vi "RVC 3-link serial robot Primatic.vi"() -> ()   [LabVIEW 2014]
uses:
  <vilib>/Analysis/Matrix/Datatypes/RealMatrix.ctl
  <vilib>/robotics/Kinematics/Analytical/Initialize Generic Serial Arm.vi
  <vilib>/robotics/Kinematics/Analytical/NI_Robotics_AnalyticKinematics.lvlib
  <vilib>/robotics/Kinematics/Robot/NI_Robotics_Serial Robot Arm.lvclass
  <vilib>/Analysis/Matrix/NI_Matrix.lvlib
panel:
  in  "appended array":dbl[](array[numeric])=[0.2, 0.2, 0.2, 0.2]
  in  "rotation angle (theta)":dbl
  in  "length (a) 2":dbl=0.3 format="%#_13g"
  in  "length (a)":dbl=0.3 format="%#_13g"
  out "transformation":picture
  out "forward kinematics":T1
  out "3D Picture":refnum<vi>(3d-picture)
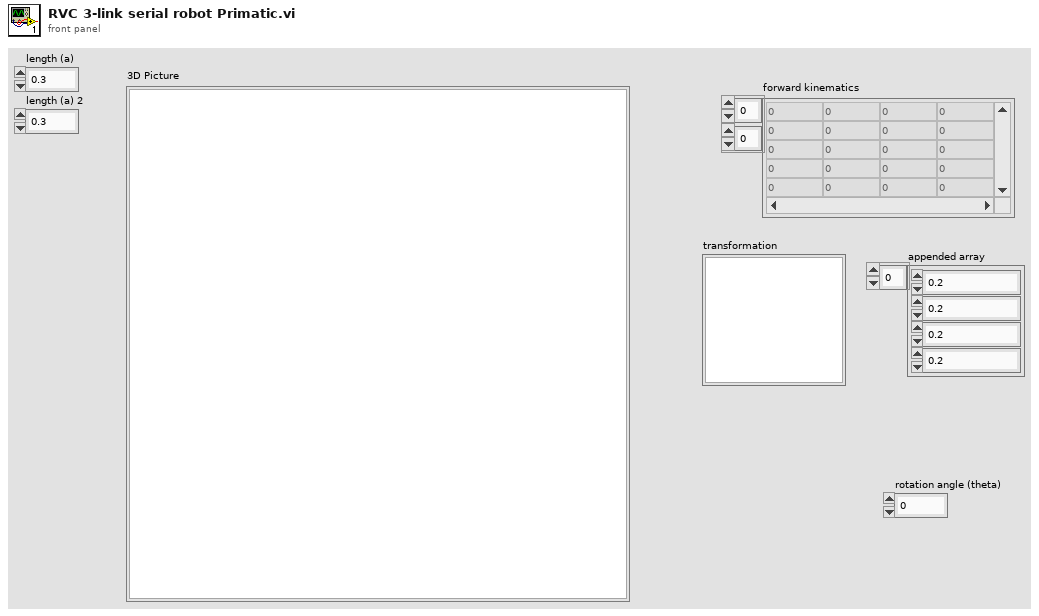
[diagram p1: front panel]
types:
  T1 = typedef "NI_Matrix.lvlib/RealMatrix.ctl" = dbl[][]
  T2 = typedef "DH Kinematic Parameters.ctl" = cluster{"twist angle":dbl, "length":dbl, "rotation angle":dbl, "offset distance":dbl, "joint type":T3, "joint coordinate offset":dbl}
  T3 = typedef "NI_Robotics_Link.lvclass/Joint Type.ctl" = enum16{"Revolute", "Prismatic"}
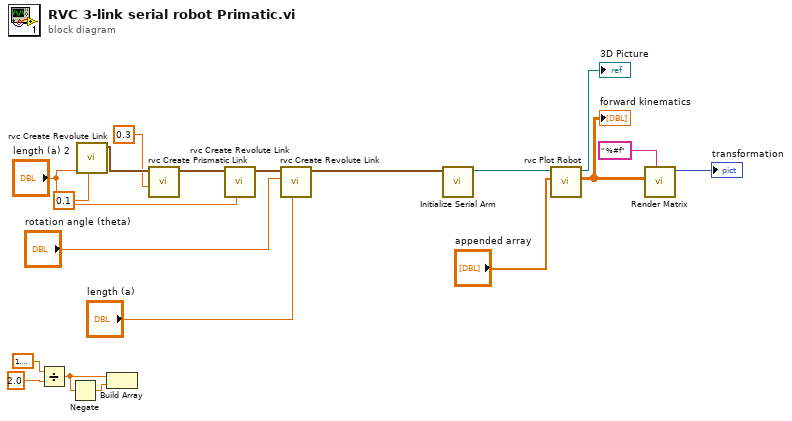
[diagram p0: block diagram]
diagram:
  n1 = Divide(x=1.5707963267948966, y=2.0) -> (x/y=w15:dbl)
  n2 = Negate(x=w15) -> (-x=w14:dbl)
  n3 = call "rvc Create Revolute Link.vi"("length (a)"=0.1, "joint coordinate offset"="length (a) 2") -> ("Array"=w4:T2[])  [unwired: 9 in]
  n4 = Build Array(w15, w14) -> ()  [unwired: 1 out]
  n5 = call "rvc Create Prismatic Link.vi"("twist angle (alpha)"=0.3 ("length (a)"), "Array 2"=w4) -> ("Array"=w5:T2[])  [unwired: 9 in]
  n6 = call "rvc Create Revolute Link.vi"("length (a)"="length (a) 2", "Array 2"=w5) -> ("Array"=w7:T2[])  [unwired: 9 in]
  n7 = call "rvc Create Revolute Link.vi"("length (a)"="length (a)", "rotation angle (theta)"="rotation angle (theta)", "Array 2"=w7) -> ("Array"=w6:T2[])  [unwired: 8 in]
  n8 = call-poly <vilib>:"Initialize Serial Arm.vi"("kinematic parameters"=w6) -> ("serial arm out"=w19:refnum<class "NI_Robotics_Serial Robot Arm.lvclass">)  [unwired: 9 in, 1 out]
  n9 = call "rvc Plot Robot.vi"("joint positions"="appended array", "NI_Robotics_Serial Robot Arm in"=w19) -> ("forward kinematics"=w10:T1, "Scene Object Out"=→"3D Picture":refnum<vi>)  [unwired: 7 in, 1 out]
  "forward kinematics" <- w10
  n10 = call "Render Matrix.vi"("format string"=" %#f", "A"=w10) -> ("picture out"=→"transformation":picture)  [unwired: 9 in]
